vi "SCT Handle Name Change.vi"(8 "error in (no error)":errorcluster caption="错误输入（无错误）", 9 "New Name":string caption="新名称", 10 "Old Name":string caption="原名称", 11 "Variable Dialog Controls in":T1 caption="变量对话控件输入") -> (0 "error out":errorcluster caption="错误输出", 3 "Variable Dialog Controls out":T1 caption="变量对话控件输出")   [LabVIEW 2016]
uses:
  <resource>/dialog/variable/SCT Variable Dialog Controls.ctl
  <vilib>/Utility/error.llb/DialogType.ctl
panel:
  in  "Duplicate Variable Name Error":string="变量名无效，名称已存在。" caption="复制变量名错误"
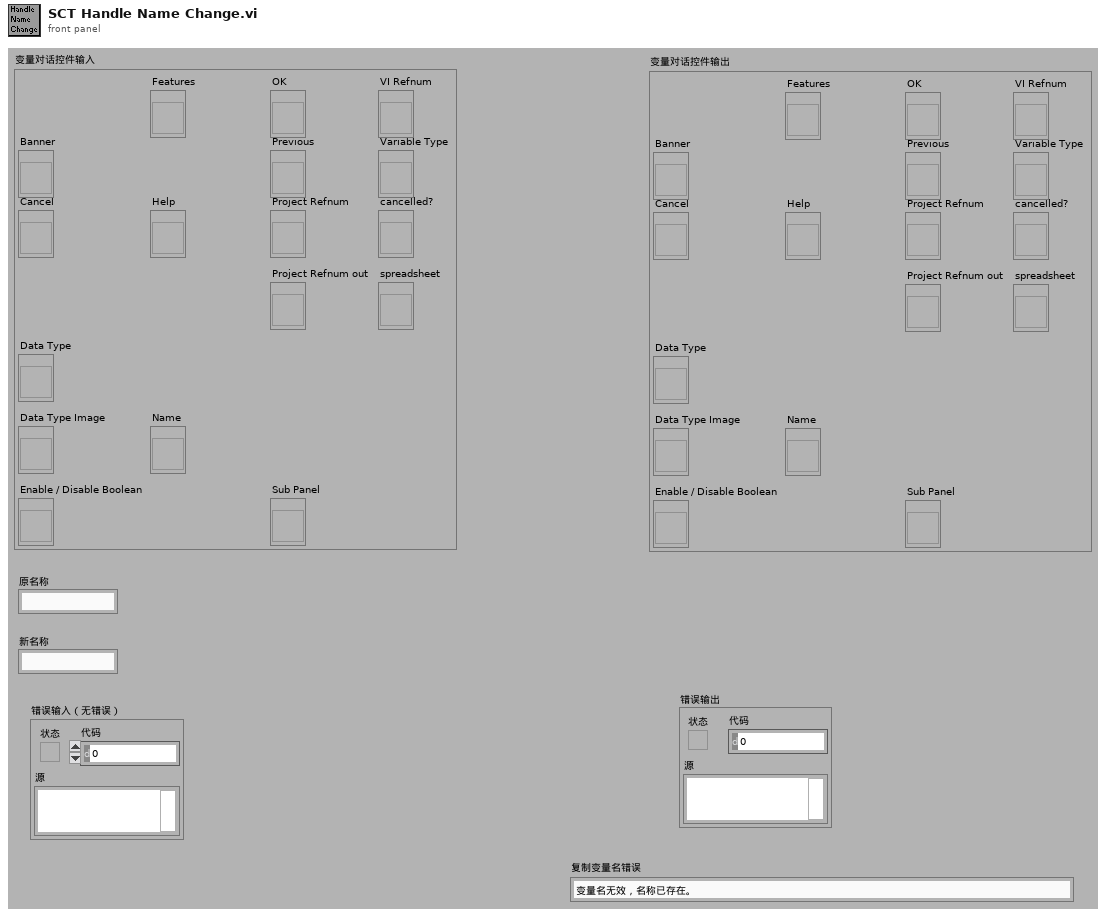
[diagram p1: front panel]
types:
  T1 = typedef "SCT Variable Dialog Controls.ctl" = cluster{"Banner":refnum<vi>, "Cancel":refnum<vi>, "Data Type":refnum<vi>, "Data Type Image":refnum<vi>, "Enable / Disable Boolean":refnum<vi>, "Features":refnum<vi>, "Help":refnum<vi>, "Name":refnum<vi>, "OK":refnum<vi>, "Previous":refnum<vi>, "Project Refnum":refnum<vi>, "Project Refnum out":refnum<vi>, "Sub Panel":refnum<vi>, "VI Refnum":refnum<vi>, "Variable Type":refnum<vi>, "cancelled?":refnum<vi>, "spreadsheet":refnum<vi>}
  T2 = typedef "DialogType.ctl" = u16
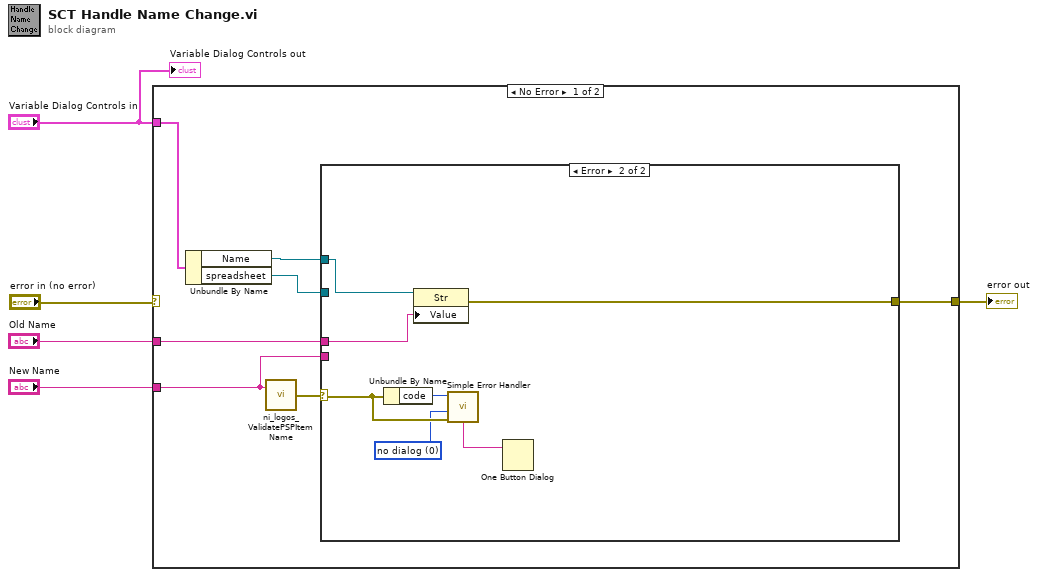
[diagram p0: block diagram]
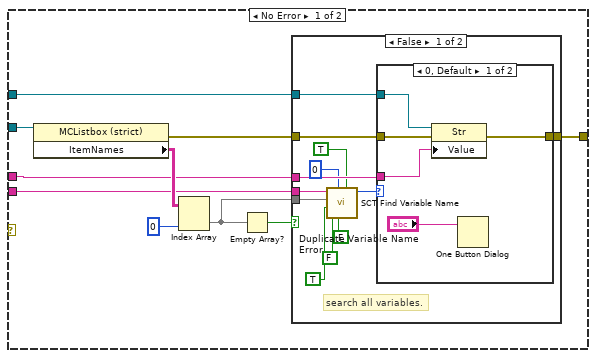
[diagram p2: hidden frame]
diagram:
  n1 = case shown="No Error" "error in (no error)" {
    selector: "error in (no error)" -> [_ w49]
    tunnel: "Variable Dialog Controls in" -> [w6 _]
    tunnel: "New Name" -> [w11 _]
    tunnel: "Old Name" -> [w10 _]
    tunnel: [w7 w49] -> w3
    frame No Error {
      n2 = Unbundle By Name(w6) -> ("Name"=w8:refnum<vi>, "spreadsheet"=w12:refnum<vi>)
      n3 = call <vilib>:"ni_logos_ValidatePSPItemName.vi"("itemName"=w11) -> ("error in(no error) 2"=w9:errorcluster)  [unwired: 1 in]
      n4 = case shown="Error" w9 {
        selector: w9 -> [_ w43]
        tunnel: w8 -> [w19 w48]
        tunnel: w10 -> [w18 w47]
        tunnel: w11 -> [w20 _]
        tunnel: w12 -> [w15 _]
        tunnel: [w13 w46] -> w7
        frame No Error {
          n5 = property on="Property Node" class="MCListbox (strict)"(reference=w15) -> (error out=w14:errorcluster, "ItemNames"=w21:string[][])  [unwired: 1 in, 1 out]
          n6 = Index Array(array=w21, index (col)=0 ("disabled index (col)")) -> (element=w17:string[])  [unwired: 1 in]
          n7 = Empty Array?(array=w17) -> (empty?=w16:bool)
          n8 = case shown="False" w16 {
            tunnel: w20 -> [w34 _]
            tunnel: w19 -> [w32 _]
            tunnel: w18 -> [w31 _]
            tunnel: w17 -> [w30 _]
            tunnel: w14 -> [w24 w41]
            tunnel: [w23 w41] -> w13
            frame False {
              # "search all variables."
              n9 = call <resource>:"SCT Find Variable Name.vi"("Find Forward"=TRUE, "RegularExpression"=FALSE, "StartIndex (0)"=0, "ExactMatchCase"=FALSE, "MatchWholeWord"=TRUE, "SearchArray"=w30, "SearchString"=w34) -> ("index (-1 = not found)"=w33:i32)  [unwired: 4 in]
              n10 = case shown="0, Default" w33 {
                tunnel: w32 -> [w39 _]
                tunnel: w31 -> [w38 _]
                tunnel: w24 -> [w36 w40]
                tunnel: [w35 w40] -> w23
                frame 0, Default {
                  n11 = property class="Str"(reference=w39, error in=w36, "Value"=w38) -> (error out=w35:errorcluster)  [unwired: 1 out]
                  n12 = One Button Dialog(message="Duplicate Variable Name Error") -> ()  [unwired: 1 in, 1 out]
                }
                frame -1 {
                }
              }
            }
            frame True {
            }
          }
        }
        frame Error {
          w42 = T2 0 items=["no dialog", "OK message", "continue or stop message", "OK message + warnings", "continue/stop + warnings"] ("type of dialog (OK msg:1)")
          n13 = Unbundle By Name(w43) -> ("code"=w45:i32)
          n14 = property class="Str"(reference=w48, "Value"=w47) -> (error out=w46:errorcluster)  [unwired: 1 in, 1 out]
          n15 = call <vilib>:"Simple Error Handler.vi"("error code (no error:0)"=w45, "type of dialog (OK msg:1)"=w42, "error in (no error)"=w43) -> ("message"=w44:string)  [unwired: 2 in, 4 out]
          n16 = One Button Dialog(message=w44) -> ()  [unwired: 1 in, 1 out]
        }
      }
    }
    frame Error {
    }
  }
  "error out" <- w3
  "Variable Dialog Controls out" <- "Variable Dialog Controls in"
